vi "Data Collection.vi"() -> ()   [LabVIEW 2014]
uses:
  <vilib>/addons/control/pid/autopid.llb/PID autotuning parameters.ctl
  <vilib>/Platform/TimedLoop/XDataNode/timing_clust.ctl
  <vilib>/Platform/TimedLoop/XDataNode/nitl_modes.ctl
  <vilib>/Platform/TimedLoop/XDataNode/wakeup.ctl
  <vilib>/FPGAPlugInAG/myRIO-1900/niLvFpga_Open_myRIO-1900.vi
  <vilib>/rvi/interface/common/dynamic/niFpgaDynamicAddResources.vi
  <vilib>/Utility/error.llb/Error Cluster From Error Code.vi
  <vilib>/rvi/errors/niLvFpgaAdjustHostInterfaceError.vi
  <vilib>/FPGAPlugInAG/Dynamic/niLvFpga_Close_Dynamic.vi
  <vilib>/Utility/file.llb/Write To Spreadsheet File (DBL).vi
  <vilib>/addons/control/pid/autopid.llb/PID Online Autotuning (Relay Feedback).vi
  <vilib>/Utility/file.llb/Write To Spreadsheet File (I64).vi
  <vilib>/rvi/interface/nirviOpenFPGA/nirviOpenFPGA.xnode
  FPGA Bitfiles/Test_FPGATarget_CurrentControl_60eBuCSPTsI.lvbitx
  Current Control.vi
  <vilib>/rvi/interface/nirviReadWriteControl/nirviReadWriteControl.xnode
  <vilib>/rvi/interface/nirviCloseFPGA/nirviCloseFPGA.xnode
  <vilib>/Platform/TimedLoop/XDataNode/XDataNode.xnode
  <vilib>/Platform/TimedLoop/XDataNode/XDNodeRunTimeDep.lvlib
  <vilib>/rvi/interface/Simulation/niFpgaSimulationCallBeginRW.vi
  <vilib>/addons/control/pid/NI_PID_autopid.lvlib
  NiFpgaLv.dll
panel:
  out "PV: Kinect Data":i32(graph)
  in  "SP in:":dbl(slide)=30.8641975308642 scale=400.0..900.0 scale format="%.1f"
  in  "PID gains in":T1={"proportional gain (Kc)"=1.0, "integral time (Ti, min)"=0.01, "derivative time (Td, min)"=0.0} {"derivative time (Td, min)" format="%.3f"; "integral time (Ti, min)" format="%.3f"; "proportional gain (Kc)" format="%.3f"}
  in  "autotuning parameters":T2={"type of controller"=0, "relay cycles"=3, "relay amplitude"=1.0, "control specifications"=2, "PV noise level"=0.1} {"PV noise level" format="%.2f"; "control specifications" items=["normal", "fast", "slow"]; "relay amplitude" format="%.2f"; "type of controller" items=["P", "PI", "PID"]}
  out "PV Out:":dbl(slide)=19.583333333333336 scale=0.0..100.0 scale format="%.1f"
  out "SP Out:":dbl(slide)=30.8641975308642 scale=0.0..100.0 scale format="%.1f"
  out "output cluster":T3
  out "Status?":bool
  out "MV: Current (mA)":i32
  out "error out":errorcluster
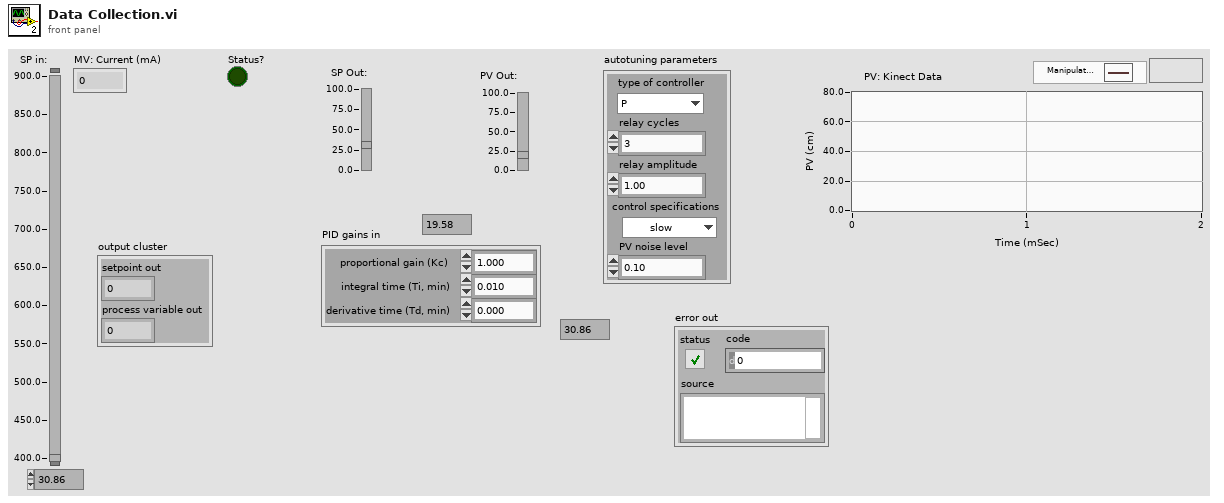
[diagram p1: front panel]
types:
  T1 = cluster{"proportional gain (Kc)":dbl, "integral time (Ti, min)":dbl, "derivative time (Td, min)":dbl}
  T2 = typedef "PID autotuning parameters.ctl" = cluster{"type of controller":u16, "relay cycles":i32, "relay amplitude":dbl, "control specifications":u16, "PV noise level":dbl}
  T3 = cluster{"setpoint out":dbl, "process variable out":dbl}
  T4 = typedef "XDNodeRunTimeDep.lvlib/timing_clust.ctl" = cluster{"Expected End [f-1]":u64, "Actual End [f-1]":u64, "Finished Late? [f-1]":bool, "Expected End [i-1]":u64, "Actual End [i-1]":u64, "Finished Late? [i-1]":bool, "Expected Start [i]":u64, "Actual Start [i]":u64, "Expected Start [f]":u64, "Actual Start [f]":u64, "Source Name":string, "Structure Name":string, "Period":i64, "Deadline":i64, "Offset":i64, "Start":i64, "Priority":i32, "Timeout":i32, "Mode":T5, "Wakeup Reason":T6, "Error":errorcluster, "Source Type":string, "Secondary Source Type":string, "Global End Time":u64, "Global Start Time":u64, "Frame Duration":u64, "Iteration Duration":u64, "Assigned CPU":i32, "I/O Scan Engine Mode":u32}
  T5 = typedef "XDNodeRunTimeDep.lvlib/nitl_modes.ctl" = enum32{"No Change", "Process missed periods, maintain original phase", "Discard missed periods, maintain original phase", "Process missed periods, ignore original phase", "Discard missed periods, ignore original phase"}
  T6 = typedef "XDNodeRunTimeDep.lvlib/wakeup.ctl" = enum32{"Normal", "Aborted", "Asynchronous wakeup", "Timing source error", "Timed loop error", "Timeout"}
  T7 = enum16{"big-endian, network order", "native, host order", "little-endian"}
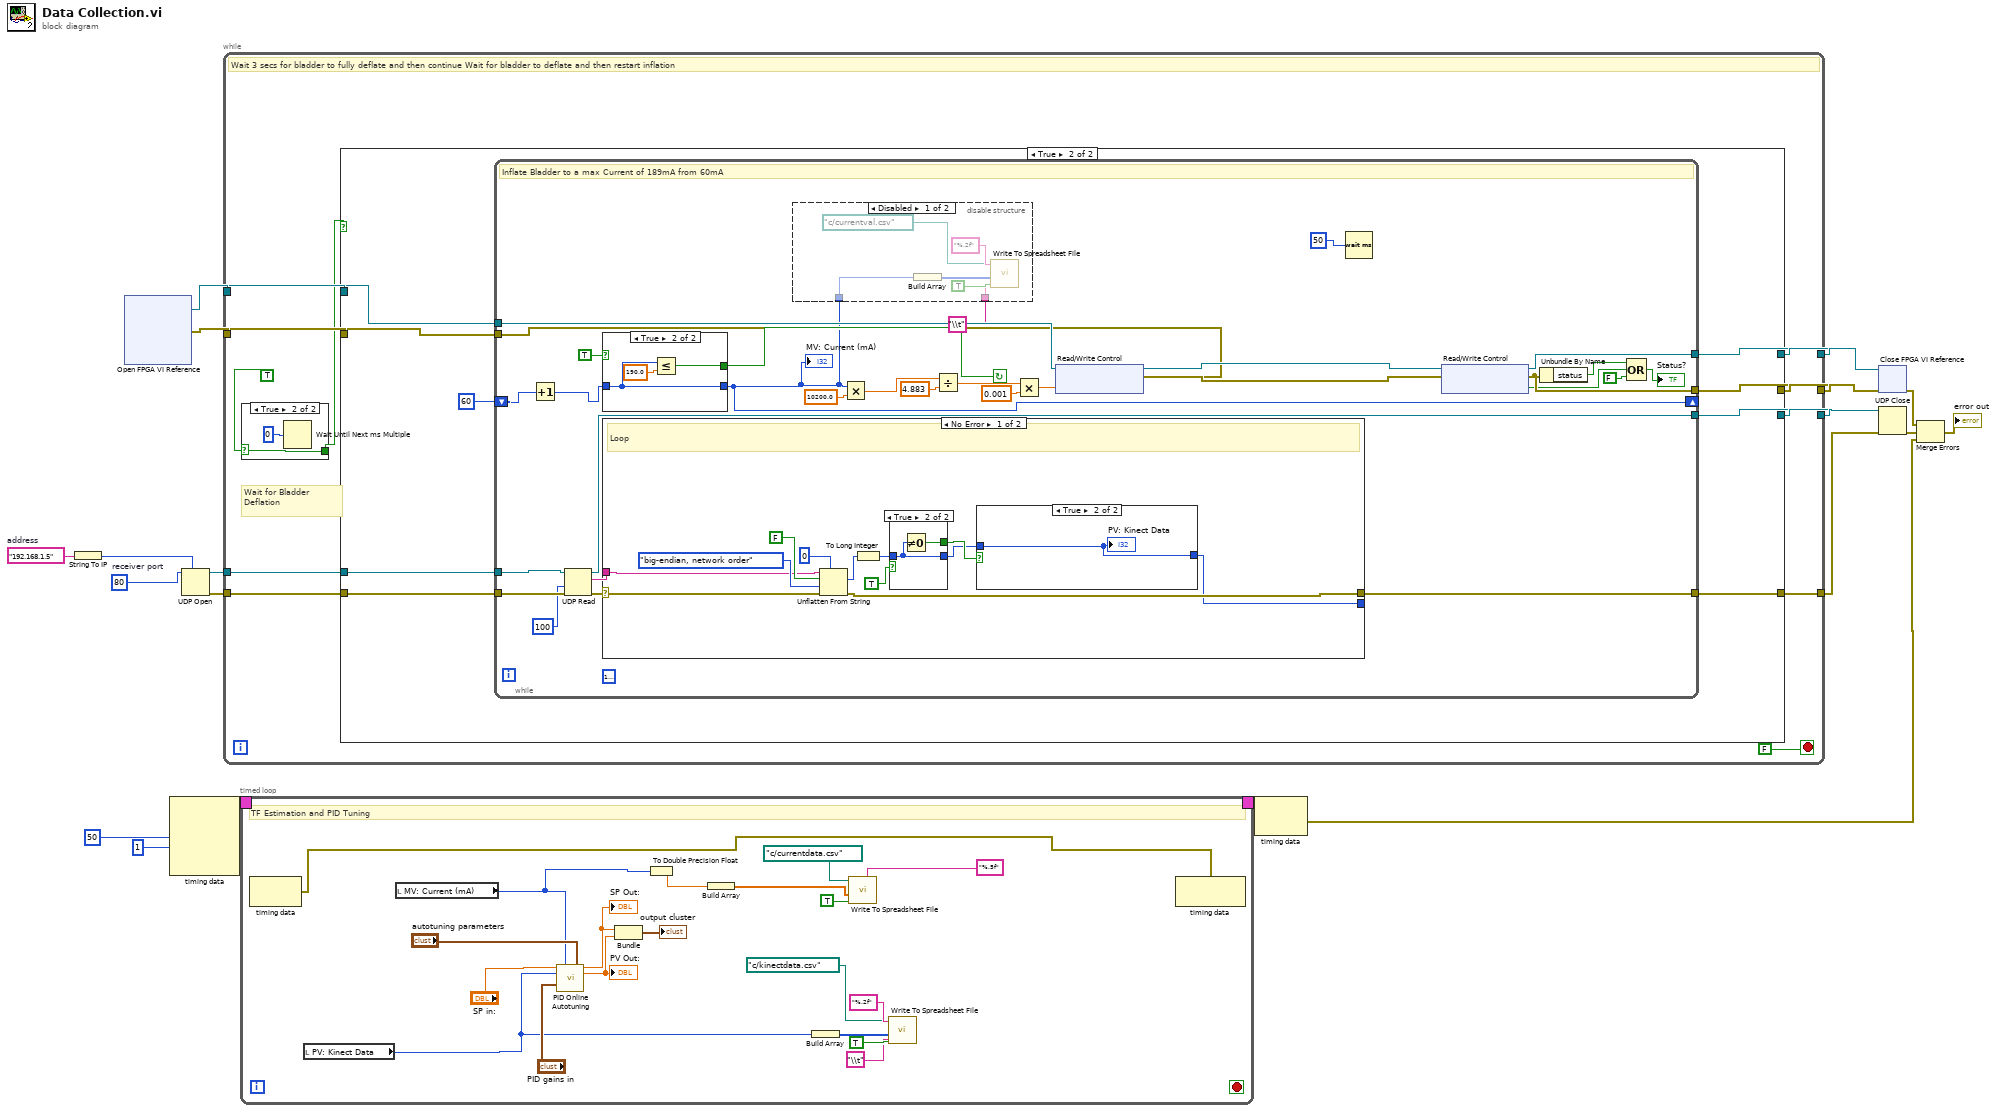
[diagram p0: block diagram]
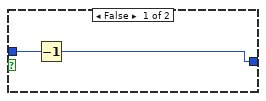
[diagram p5: hidden frame]
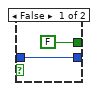
[diagram p6: hidden frame]
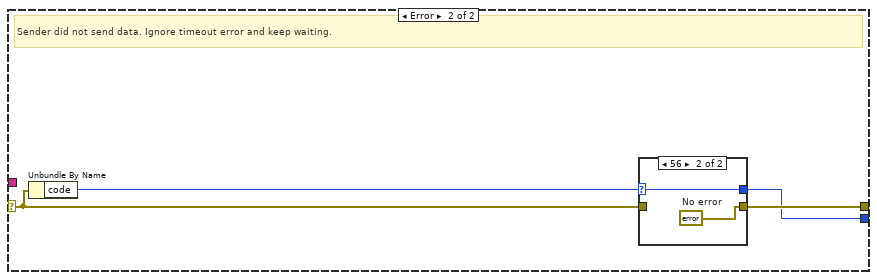
[diagram p7: hidden frame]
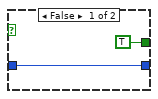
[diagram p9: hidden frame]
diagram:
  w16 = "192.168.1.5"  # address
  w15 = u16 80  # receiver port
  n1 = String To IP(1:w16) -> (0:w17:u32)
  n2 = xnode "Open FPGA VI Reference"() -> ("FPGA VI Reference Out"=w5:refnum<k20>, "error out"=w8:errorcluster)  [unwired: 2 in]
  n3 = node-c288(i64 50 ("Period"), 1 ("Processor")) -> (w19:T4)  [unwired: 2 in]
  n4 = UDP Open(7:w17, 11:w15) -> (port=w14:refnum<k16>, 0:w13:errorcluster)  [unwired: 3 in, 1 out]
  n5 = while {
    tunnel: w5 -> [w24]
    tunnel: [w25] -> w6
    tunnel: w8 -> [w27]
    tunnel: [w26] -> w7
    tunnel: w14 -> [w30]
    tunnel: [w28] -> w12
    tunnel: w13 -> [w29]
    tunnel: [w21] -> w3
    stop <- FALSE stop-if-true
    # "Wait for Bladder Deflation"
    # "Wait 3 secs for bladder to fully deflate and then continue Wait for bladder to deflate and then restart inflation"
    n6 = case shown="True" TRUE {
      selector: TRUE -> [w31 w32]
      tunnel: [w31 w32] -> w22
      frame False {
      }
      frame True {
        n7 = Wait Until Next ms Multiple(millisecond multiple=u32 0) -> ()  [unwired: 1 out]
      }
    }
    n8 = case shown="True" w22 {
      tunnel: w30 -> [w35 w46]
      tunnel: w29 -> [w34 w45]
      tunnel: [w35 w44] -> w28
      tunnel: w27 -> [w36 w43]
      tunnel: [w36 w42] -> w26
      tunnel: [w37 w41] -> w25
      tunnel: w24 -> [w37 w40]
      tunnel: [w34 w38] -> w21
      frame False {
      }
      frame True {
        n9 = while {
          tunnel: w46 -> [w76]
          tunnel: [w74] -> w44
          tunnel: w45 -> [w75]
          tunnel: w40 -> [w70]
          tunnel: [w71] -> w41
          tunnel: w43 -> [w52]
          tunnel: [w72] -> w42
          shift-right: [w50] -> _
          shift-left: 60 -> [w48]
          tunnel: [w53] -> w38
          stop <- w56 continue-if-true
          (unwired) u32 16777216
          # "Inflate Bladder to a max Current of 189mA from 60mA"
          n10 = Increment(x=w48) -> (x+1=w47:i32)
          n11 = UDP Read(connection ID=w76, timeout ms (25000)=100, 8:w75) -> (data out=w55:string, error out=w54:errorcluster, 3:w74:refnum<k16>)  [unwired: 3 out]
          n12 = case shown="True" TRUE {
            tunnel: w47 -> [w111 w112]
            tunnel: [TRUE w113] -> w56
            tunnel: [w111 w112] -> w50
            frame False {
            }
            frame True {
              n13 = Less Or Equal?(x=w112, y=190.0) -> (x <= y?=w113:bool)
            }
          }
          "MV: Current (mA)" <- w50
          n14 = case shown="No Error" w54 {
            selector: w54 -> [w89 w104]
            tunnel: w55 -> [w90 _]
            tunnel: [w88 w103] -> w53
            tunnel: [w83 w102] -> _
            frame No Error {
              # "Loop"
              n15 = Unflatten From String(type=0, binary string=w90, data includes array or string size? (T)=FALSE, byte order (0:big-endian, network order)=T7."big-endian, network order" ("byte order"), error in (no error)=w89) -> (value=w91:i32, error out=w88:errorcluster)  [unwired: 1 out]
              n16 = To Long Integer(number=w91) -> (32bit integer=w86:i32)
              n17 = case shown="True" TRUE {
                tunnel: w86 -> [w98 w100]
                tunnel: [FALSE w101] -> w85
                tunnel: [w98 w100] -> w84
                frame False {
                }
                frame True {
                  n18 = Not Equal To 0?(x=w100) -> (x != 0?=w101:bool)
                }
              }
              n19 = case shown="True" w85 {
                tunnel: w84 -> [w96 w97]
                tunnel: [w95 w97] -> w83
                frame False {
                  n20 = Decrement(x=w96) -> (x-1=w95:i32)
                }
                frame True {
                  "PV: Kinect Data" <- w97
                }
              }
            }
            frame Error {
              # "Sender did not send data. Ignore timeout error and keep waiting."
              n21 = Unbundle By Name(w104) -> ("code"=w105:i32)
              n22 = case shown="56" w105 {
                selector: w105 -> [w106 w108]
                tunnel: w104 -> [w107 _]
                tunnel: [w107 w109] -> w103
                tunnel: [w106 w108] -> w102
                frame Default {
                }
                frame 56 {
                  w109 = errorcluster {"status"=FALSE, "code"=0, "source"=""}  # No error
                }
              }
            }
          }
          n23 = disable-structure shown="Disabled" {
            disable-tunnel: "\\t" ("delimiter (\\t)") -> [w80 _]
            disable-tunnel: w50 -> [w77 _]
            frame Disabled {
              n24 = Build Array(w77) -> (w82:i32[])
              n25 = call-poly <vilib>:"Write To Spreadsheet File.vi"("delimiter (\\t)"=w80, "format (%d)"="%.2f", "append to file? (new file:F)"=TRUE, "1D data"=w82, "file path (dialog if empty)"=path "c:/currentval.csv") -> ()  [unwired: 3 in, 1 out]
            }
            frame Enabled {
            }
          }
          n26 = Multiply(x=w50, y=10200.0) -> (x*y=w58:dbl)
          n27 = Divide(x=w58, y=4.883) -> (x/y=w61:dbl)
          n28 = Multiply(x=w61, y=0.001) -> (x*y=w67:dbl)
          n29 = xnode "Read/Write Control"("FPGA VI Reference In"=w70, "error in"=w52, "DAC Inlet Valve"=w67) -> ("FPGA VI Reference Out"=w69:refnum<k20>, "error out"=w68:errorcluster)
          n30 = Wait (ms)(milliseconds to wait=i64 50 ("Period")) -> ()  [unwired: 1 out]
          n31 = xnode "Read/Write Control"("FPGA VI Reference In"=w69, "error in"=w68) -> ("FPGA VI Reference Out"=w71:refnum<k20>, "error out"=w72:errorcluster, "Inlet Overflow?"=w66:bool)
          n32 = Unbundle By Name(w72) -> ("status"=w64:bool)
          n33 = Compound Arithmetic op=OR(w64, w66, FALSE ("value")) -> (→"Status?":bool)
        }
      }
    }
  }
  n34 = timed-loop {
    timing: w19 -> [_]
    timing-out: [_] -> w18
    stop <- _ stop-if-true
    # "TF Estimation and PID Tuning"
    n35 = node-c288() -> (w122:errorcluster)  [unwired: 1 in]
    n36 = local read "PV: Kinect Data"() -> (w115:i32)
    n37 = local read "MV: Current (mA)"() -> (w127:i32)
    n38 = call-poly <vilib>:"PID Online Autotuning.vi"("setpoint"="SP in:", "manipulated variable"=w127, "autotuning parameters"="autotuning parameters", "process variable"=w115, "PID gains in"="PID gains in") -> ("setpoint out"=w130:dbl, "process variable out"=w129:dbl)  [unwired: 6 in, 3 out]
    "PV Out:" <- w129
    "SP Out:" <- w130
    n39 = Bundle("setpoint out"=w130, "process variable out"=w129) -> (→"output cluster":T3)  [unwired: 1 in]
    n40 = To Double Precision Float(number=w127) -> (double precision float=w126:dbl)
    n41 = Build Array(w126) -> (w121:dbl[])
    n42 = Build Array(w115) -> (w120:i32[])
    n43 = call-poly <vilib>:"Write To Spreadsheet File.vi"("format (%.3f)"="%.5f", "append to file? (new file:F)"=TRUE, "1D data"=w121, "file path (dialog if empty)"=path "c:/currentdata.csv") -> ()  [unwired: 4 in, 1 out]
    n44 = call-poly <vilib>:"Write To Spreadsheet File.vi"("delimiter (\\t)"="\\t" ("delimiter (\\t)"), "format (%d)"="%.2f", "append to file? (new file:F)"=TRUE, "1D data"=w120, "file path (dialog if empty)"=path "c:/kinectdata.csv") -> ()  [unwired: 3 in, 1 out]
    n45 = node-c288(w122) -> ()  [unwired: 1 out]
  }
  n46 = node-c288(w18) -> (w1:errorcluster)
  n47 = xnode "Close FPGA VI Reference"("FPGA VI Reference In"=w6, "error in"=w7) -> ("error out"=w9:errorcluster)
  n48 = UDP Close(connection ID=w12, 8:w3) -> (error out=w11:errorcluster)  [unwired: 1 out]
  n49 = Merge Errors(w9, w11, w1) -> (→"error out":errorcluster)
